vi "限幅器（TimeStamp）.vi"(3 "下限":timestamp, 4 "X_in":timestamp, 5 "上限":timestamp) -> (1 "X_Out":timestamp)   [LabVIEW 2012]
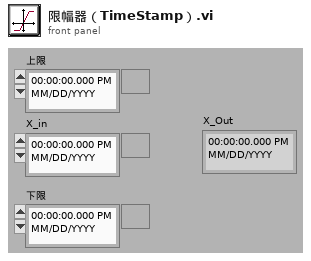
[diagram p1: front panel]
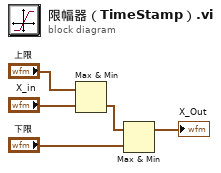
[diagram p0: block diagram]
diagram:
  n1 = Max & Min(x="上限", y="X_in") -> (min(x,y)=w3:timestamp)  [unwired: 1 out]
  n2 = Max & Min(x=w3, y="下限") -> (max(x,y)=→"X_Out":timestamp)  [unwired: 1 out]
